vi "pointer.condition.null.vi"(7 "Pointer methods":T1, 8 "error in (no error)":errorcluster, 11 "TestCase in":refnum<class "TestCase.Pointer.lvclass">) -> (0 "error out":errorcluster, 3 "TestCase out":refnum<class "TestCase.Pointer.lvclass">)   [LabVIEW 2016, in "TestCase.Pointer.lvclass"]
uses:
  TestCase.Pointer.lvclass
  pointer methods.ctl
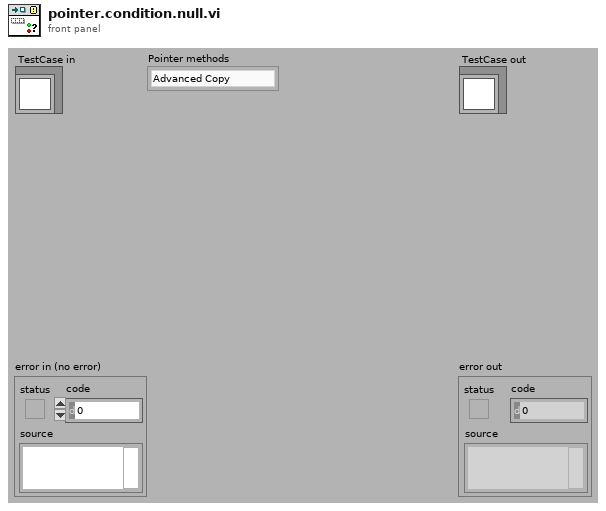
[diagram p1: front panel]
types:
  T1 = typedef "TestCase.Pointer.lvclass/pointer methods.ctl" = enum16{"Advanced Copy", "Check If Equal Size", "Check If Equal Contents", "Check", "Clear Subset", "Clear", "Copy All", "Copy", "Duplicate", "Read", "Swap", "Write"}
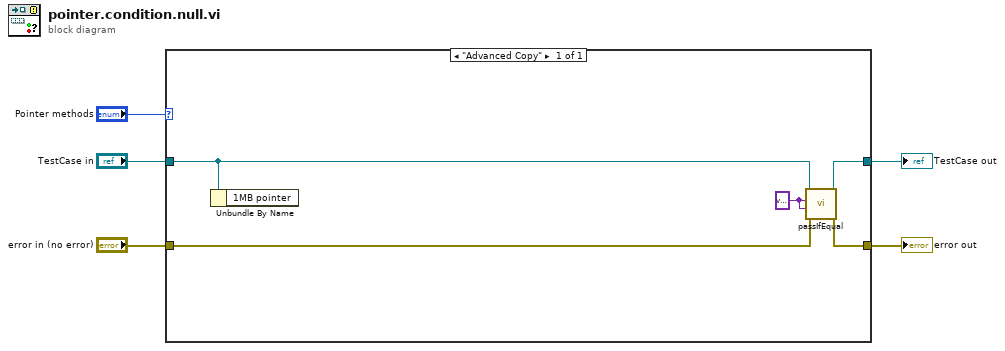
[diagram p0: block diagram]
diagram:
  n1 = case shown="\"Advanced Copy\"" "Pointer methods" {
    tunnel: "error in (no error)" -> [w10]
    tunnel: [w9] -> w4
    tunnel: "TestCase in" -> [w6]
    tunnel: [w8] -> w2
    frame "Advanced Copy" {
      w7 = variant ("x")
      n2 = Unbundle By Name(w6) -> ()  [unwired: 1 out]
      n3 = call-dynamic "passIfEqual.vi"("error in (no error)"=w10, "y"=w7, "x"=w7, "TestCase in"=w6) -> ("error out"=w9:errorcluster, "TestCase out"=w8:refnum<class "TestCase.Pointer.lvclass">)  [unwired: 6 in]
    }
  }
  "error out" <- w4
  "TestCase out" <- w2
